vi "Get Temperature Status.vi"(0 "SensorTemp":sgl, 5 "TargetTemp":sgl, 7 "AmbientTemp":sgl, 9 "CoolerVolts":sgl, 11 "error in (no error)":errorcluster) -> (3 "function return":u32, 4 "SensorTemp out":sgl, 6 "TargetTemp out":sgl, 8 "AmbientTemp out":sgl, 10 "CoolerVolts out":sgl, 15 "error out":errorcluster)   [LabVIEW 2014, in "atmcd32d.lvlib"]
doc: "unsigned int WINAPI GetTemperatureStatus(float * SensorTemp, float * TargetTemp, float * AmbientTemp, float * CoolerVolts);"
uses:
  atmcd32d.lvlib
  atmcd32d.dll
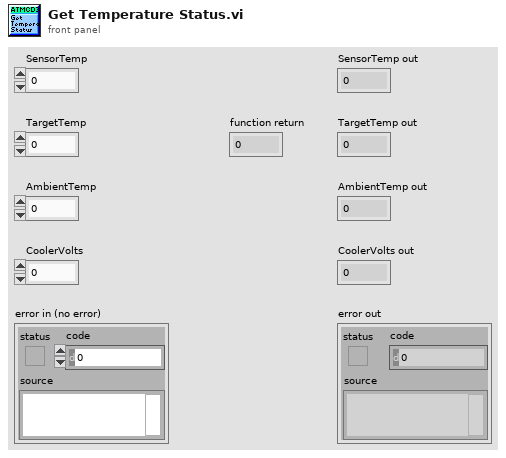
[diagram p1: front panel]
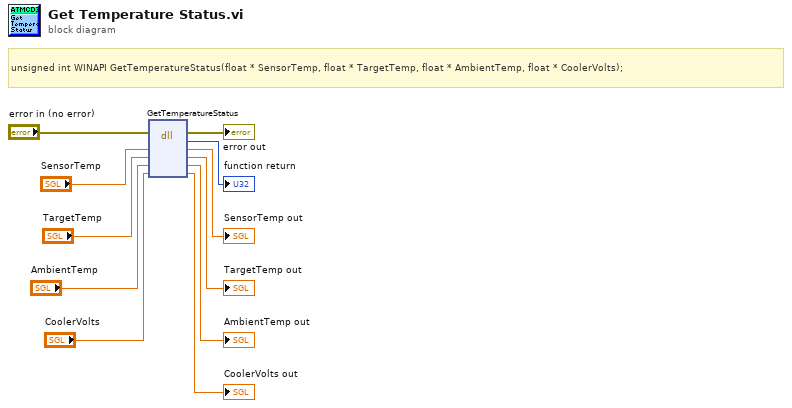
[diagram p0: block diagram]
diagram:
  # "unsigned int WINAPI GetTemperatureStatus(float * SensorTemp, float * TargetTemp, float * AmbientTemp, float * CoolerVolts);"
  n1 = dll-call lib="C:/Users/Bakir/Documents/Lambda2-Testing/lib/Andorlib/atmcd32d.*" fn="GetTemperatureStatus"(error in="error in (no error)", "SensorTemp"="SensorTemp", "TargetTemp"="TargetTemp", "AmbientTemp"="AmbientTemp", "CoolerVolts"="CoolerVolts") -> (error out=→"error out":errorcluster, →"function return":u32, "SensorTemp"=→"SensorTemp out":sgl, "TargetTemp"=→"TargetTemp out":sgl, "AmbientTemp"=→"AmbientTemp out":sgl, "CoolerVolts"=→"CoolerVolts out":sgl)  [unwired: 2 in, 1 out]
